vi "Setup voltage in.vi"(7 "error in (no error)":errorcluster, 10 "Sampling info in":T1={"Channels"=[], "Sampling freq"=0.0, "Output freq"=0.0, "Update freq"=0.0, "Steps per rev"=0, "Counts per rev"=0, "Amplifier"="", "Motor driver"="", "Step bit"=0, "Max speed"=0.0, "Max accel"=0.0, "Pos gain"=0.0, "Vel gain"=0.0, "counter"="Dev1/ctr0"} {"Channels"."Hi cutoff" items=["500"=500.0, "1k"=1000.0, "5k"=5000.0, "10k"=10000.0, "20k"=20000.0]; "Channels"."Lo cutoff" items=["0.1"=0.1, "1"=1.0, "10"=10.0, "100"=100.0, "300"=300.0]; "Channels"."Gain" items=["x100"=100, "x1000"=1000, "x10000"=10000]}) -> (0 "error out":errorcluster, 1 "number of input samples":i32, 2 "update period":dbl, 3 "task out":refnum<k21>)   [LabVIEW 2013]
uses:
  Sampling info.ctl
  Channel.ctl
  <vilib>/DAQmx/configure/timing.llb/DAQmx Timing (Sample Clock).vi
  <vilib>/DAQmx/create/channels.llb/DAQmx Create Channel (AI-Voltage-Basic).vi
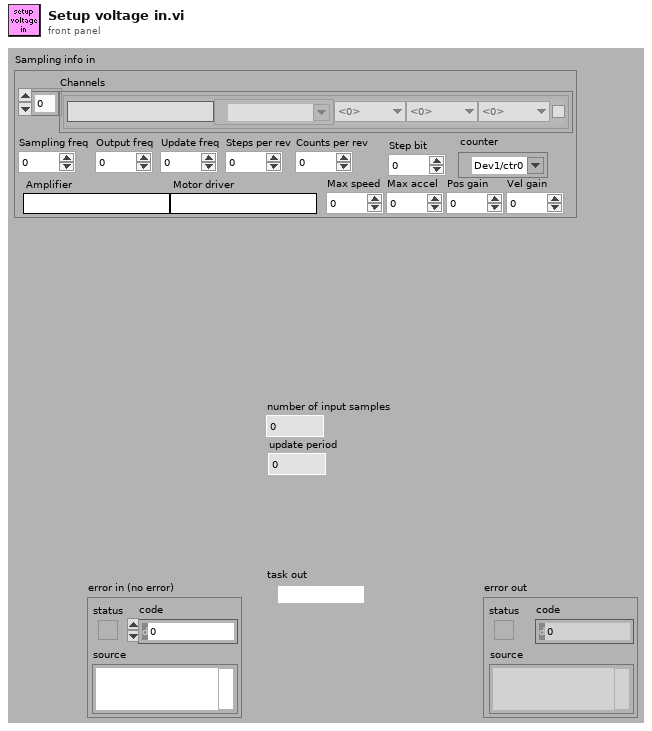
[diagram p1: front panel]
types:
  T1 = typedef "Sampling info.ctl" = cluster{"Channels":T2[], "Sampling freq":dbl, "Output freq":dbl, "Update freq":dbl, "Steps per rev":i32, "Counts per rev":i32, "Amplifier":string, "Motor driver":string, "Step bit":u8, "Max speed":dbl, "Max accel":dbl, "Pos gain":dbl, "Vel gain":dbl, "counter":tag}
  T2 = typedef "Channel.ctl" = cluster{"Name":string, "Chan":tag, "Gain":u16, "Lo cutoff":dbl, "Hi cutoff":dbl, "Notch":bool}
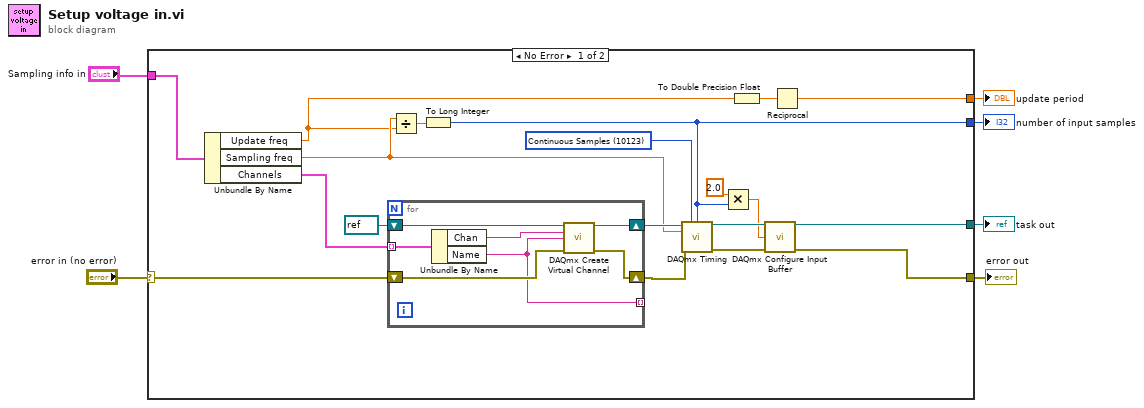
[diagram p0: block diagram]
diagram:
  n1 = case shown="No Error" "error in (no error)" {
    selector: "error in (no error)" -> [w23 w33]
    tunnel: [w13 w33] -> w5
    tunnel: "Sampling info in" -> [w24 _]
    tunnel: [w12 _] -> w3
    tunnel: [w11 _] -> w2
    tunnel: [w8 _] -> w1
    frame No Error {
      w19 = 10123 items=["Finite Samples"=10178, "Continuous Samples"=10123, "Hardware Timed Single Point"=12522] ("sample mode")
      n2 = Unbundle By Name(w24) -> ("Update freq"=w7:dbl, "Sampling freq"=w10:dbl, "Channels"=w22:T2[])
      n3 = for {
        tunnel: w22 -> [w32] mode=indexing
        shift-right: [w31] -> w21
        shift-left: refnum<k21> refnum ("task out") -> [w30]
        shift-right: [w27] -> w20
        shift-left: w23 -> [w28]
        tunnel: [w26] -> _ mode=indexing
        n4 = Unbundle By Name(w32) -> ("Chan"=w29:tag, "Name"=w26:string)
        n5 = call-poly <vilib>:"DAQmx Create Virtual Channel.vi"("task in"=w30, "physical channels"=w29, "name to assign"=w26, "error in"=w28) -> ("task out"=w31:refnum<k21>, "error out"=w27:errorcluster)  [unwired: 5 in, 5 out]
      }
      n6 = Divide(x=w10, y=w7) -> (x/y=w18:dbl)
      n7 = To Long Integer(number=w18) -> (32bit integer=w11:i32)
      n8 = call-poly <vilib>:"DAQmx Timing.vi"("task/channels in"=w21, "sample mode"=w19, "samples per channel"=w11, "rate"=w10, "error in"=w20) -> ("task out"=w17:refnum<k21>, "error out"=w16:errorcluster)  [unwired: 9 in]
      n9 = Multiply(x=2.0, y=w11) -> (x*y=w14:dbl)
      n10 = To Double Precision Float(number=w7) -> (double precision float=w9:dbl)
      n11 = call <vilib>:"DAQmx Configure Input Buffer.vi"("task/channels in"=w17, "buffer size (in samples per channel)"=w14, "error in"=w16) -> ("task out"=w12:refnum<k21>, "error out"=w13:errorcluster)  [unwired: 11 in]
      n12 = Reciprocal(x=w9) -> (1/x=w8:dbl)
    }
    frame Error {
    }
  }
  "error out" <- w5
  "task out" <- w3
  "number of input samples" <- w2
  "update period" <- w1
